vi "Ammeter Test Communications.vi"(8 "error in (no error)":errorcluster, 11 "VISA resource name in":refnum<visa-resource-name>) -> (0 "error out":errorcluster, 3 "VISA resource name out":refnum<visa-resource-name>)   [LabVIEW 2016, in "Hall Effect Library.lvlib"]
uses:
  Hall Effect Library.lvlib
  Global Variables/Instruments.vi
  Ammeter Test Communications (None).vi
  Ammeter Test Communications (648X).vi
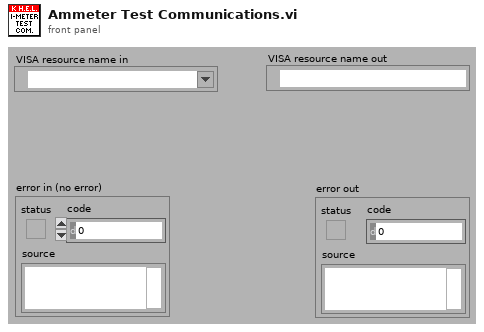
[diagram p1: front panel]
types:
  T1 = typedef "Hall Effect Library.lvlib/Ammeters.ctl" = enum16{"None", "648X"}
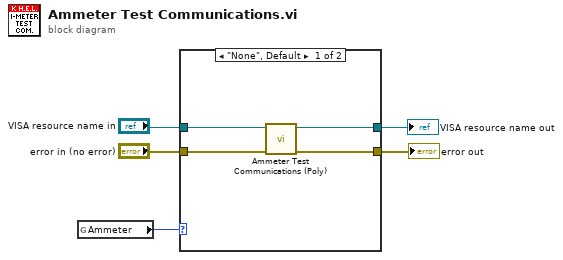
[diagram p0: block diagram]
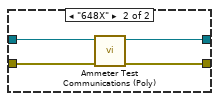
[diagram p2: hidden frame]
diagram:
  n1 = global read "Instruments.vi" "Ammeter"() -> (w5:T1)
  n2 = case shown="\"None\", Default" w5 {
    tunnel: "VISA resource name in" -> [w9 w13]
    tunnel: "error in (no error)" -> [w8 w12]
    tunnel: [w7 w11] -> w1
    tunnel: [w6 w10] -> w2
    frame "None", Default {
      n3 = call-poly "Ammeter Test Communications (Poly).vi"("error in (no error)"=w8, "VISA resource name in"=w9) -> ("error out"=w7:errorcluster, "VISA resource name out"=w6:refnum<visa-resource-name>)  [unwired: 8 out]
    }
    frame "648X" {
      n4 = call-poly "Ammeter Test Communications (Poly).vi"("error in (no error)"=w12, "VISA resource name in"=w13) -> ("error out"=w11:errorcluster, "VISA resource name out"=w10:refnum<visa-resource-name>)  [unwired: 8 out]
    }
  }
  "error out" <- w1
  "VISA resource name out" <- w2
